vi "Gyro Drive Forward.vi"(3 "Enable?":bool, 4 "Y":dbl, 5 "X":dbl, 6 "Gyro Name":string="My Gyro RefNum") -> (0 "Y out":dbl, 1 "X out":dbl, 2 "Enabled?":bool)   [LabVIEW 2013]
uses:
  <vilib>/addons/control/pid/pid.llb/PID (DBL).vi
  <vilib>/addons/control/pid/NI_PID_pid.lvlib
panel:
  out "Angle":dbl
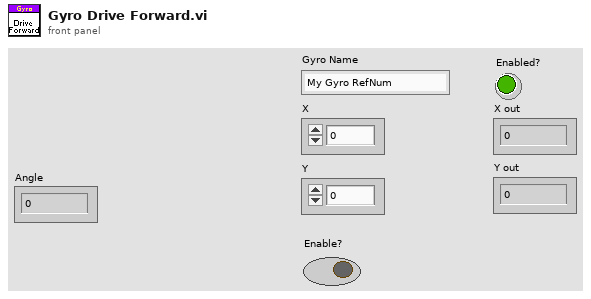
[diagram p1: front panel]
types:
  T1 = cluster{"proportional gain (Kc)":dbl, "integral time (Ti, min)":dbl, "derivative time (Td, min)":dbl}
  T2 = typedef "WPI_GyroDevRef.ctl" = cluster{"DevStatus":errorcluster, "Analog Module":T3, "Analog Channel":T4, "Offset":dbl, "Gain (VoltsPerDegree/Second)":dbl}
  T3 = typedef "FPGA_TypedefAnalogModule.ctl" = enum16{"Analog Module 1", "Analog Module 2"}
  T4 = typedef "FPGA_AIChannel.ctl" = enum8{"AI 1", "AI 2", "AI 3", "AI 4", "AI 5", "AI 6", "AI 7", "AI 8", "Invalid"}
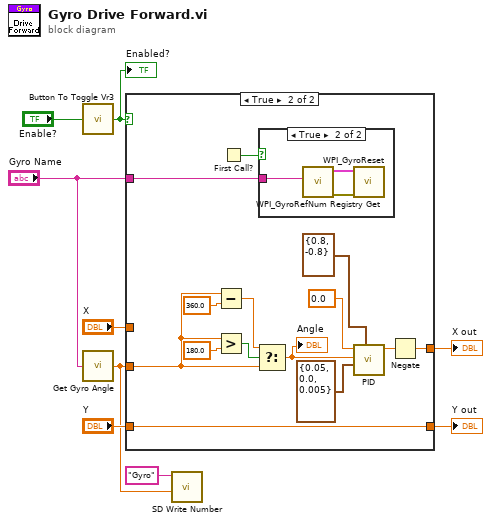
[diagram p0: block diagram]
diagram:
  n1 = call "Button To Toggle Vr3.vi"("InValue"="Enable?") -> ("Result"=w2:bool)
  "Enabled?" <- w2
  n2 = call "Get Gyro Angle.vi"("refnum name"="Gyro Name") -> ("Angle"=w1:dbl)
  n3 = case shown="True" w2 {
    tunnel: [w11 w15] -> w9
    tunnel: "Y" -> [w11 w15]
    tunnel: "X" -> [w10 _]
    tunnel: [w10 w16] -> w6
    tunnel: w1 -> [_ w14]
    tunnel: "Gyro Name" -> [_ w12]
    frame False {
    }
    frame True {
      n4 = Subtract(x=w14, y=360.0) -> (x-y=w22:dbl)
      n5 = Greater?(x=w14, y=180.0) -> (0:w21:bool)
      n6 = First Call?() -> (First Call?: T/F=w13:bool)
      n7 = Select(t=w22, s=w21, f=w14) -> (s? t:f=w17:dbl)
      "Angle" <- w17
      n8 = case shown="True" w13 {
        tunnel: w12 -> [_ w26]
        frame False {
        }
        frame True {
          n9 = call <vilib>:"WPI_GyroRefNum Registry Get.vi"("refnum name"=w26) -> ("error out"=w28:errorcluster, "GyroDevRef"=w27:T2)  [unwired: 9 in]
          n10 = call <vilib>:"WPI_GyroReset.vi"("error in (no error)"=w28, "GyroDevRef"=w27) -> ()  [unwired: 8 in, 2 out]
        }
      }
      n11 = call-poly <vilib>:"PID.vi"("output range"=cluster{"output high":dbl, "output low":dbl} {"output high"=0.8, "output low"=-0.8}, "PID gains"=T1 {"proportional gain (Kc)"=0.05, "integral time (Ti, min)"=0.0, "derivative time (Td, min)"=0.005}, "process variable"=w17, "setpoint"=0.0) -> ("output"=w23:dbl)  [unwired: 6 in, 1 out]
      n12 = Negate(x=w23) -> (-x=w16:dbl)
    }
  }
  "X out" <- w6
  "Y out" <- w9
  n13 = call <vilib>:"SD Write Number.vi"("Numeric"=w1, "Name"="Gyro") -> ()  [unwired: 8 in, 2 out]
